vi "UpdateDialog.vi"(8 "error in (no error)":errorcluster, 9 "Engine in":refnum<class "Engine.lvclass">, 11 "Highscore in":refnum<class "HighscoreDialog.lvclass">) -> (0 "error out":errorcluster, 1 "Engine out":refnum<class "Engine.lvclass">, 3 "Highscore out":refnum<class "HighscoreDialog.lvclass">)   [LabVIEW 2019, in "RT_Game.lvlib" / "HighscoreDialog.lvclass"]
uses:
  HighscoreDialog.lvclass
  C:/Users/FreshBob/Dropbox/VIs/myRIO_GameConsole/RT/RT_Game/GameObject/GameObject.lvclass
  Engine/Engine.lvclass
  GameObject/GameObject.lvclass/GameObject.ctl
  GameObject/Read IsActive.vi
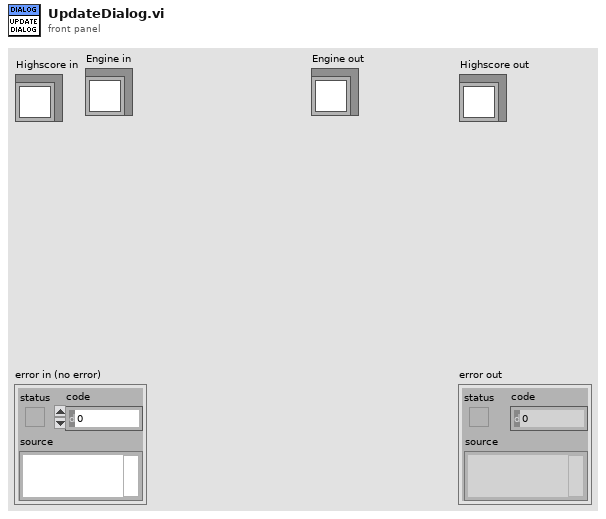
[diagram p1: front panel]
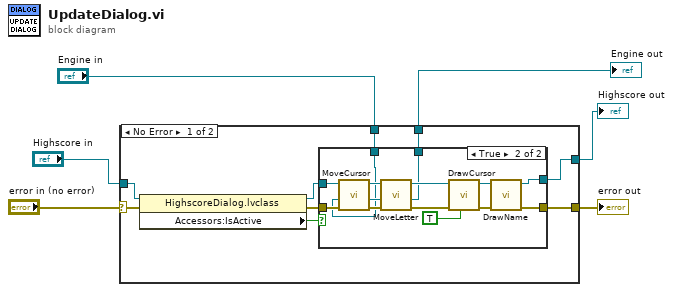
[diagram p0: block diagram]
diagram:
  n1 = case shown="No Error" "error in (no error)" {
    selector: "error in (no error)" -> [w15 w35]
    tunnel: [w13 w35] -> w5
    tunnel: [w14 w34] -> w3
    tunnel: "Highscore in" -> [w11 w34]
    tunnel: "Engine in" -> [w8 w33]
    tunnel: [w7 w33] -> w1
    frame No Error {
      n2 = property class="HighscoreDialog.lvclass"(reference=w11, error in=w15) -> (reference out=w10:refnum<class "HighscoreDialog.lvclass">, error out=w12:errorcluster, "Accessors:IsActive"=w9:bool)
      n3 = case shown="True" w9 {
        tunnel: w12 -> [w17 w32]
        tunnel: w10 -> [w18 w30]
        tunnel: [w18 w23] -> w14
        tunnel: [w17 w22] -> w13
        tunnel: w8 -> [w16 w19]
        tunnel: [w16 w21] -> w7
        frame False {
        }
        frame True {
          n4 = call "MoveCursor.vi"("error in (no error)"=w32, "Engine in"=w19, "Highscore in"=w30) -> ("error out"=w31:errorcluster, "Engine out"=w20:refnum<class "Engine.lvclass">, "Highscore out"=w28:refnum<class "HighscoreDialog.lvclass">)  [unwired: 6 in]
          n5 = call "MoveLetter.vi"("error in (no error)"=w31, "Engine in"=w20, "Highscore in"=w28) -> ("error out"=w29:errorcluster, "Engine out"=w21:refnum<class "Engine.lvclass">, "Highscore out"=w26:refnum<class "HighscoreDialog.lvclass">)  [unwired: 6 in]
          n6 = call "DrawCursor.vi"("Visible?"=TRUE, "error in (no error)"=w29, "Highscore in"=w26) -> ("error out"=w27:errorcluster, "Highscore out"=w24:refnum<class "HighscoreDialog.lvclass">)  [unwired: 7 in]
          n7 = call "DrawName.vi"("error in (no error)"=w27, "Highscore in"=w24) -> ("error out"=w22:errorcluster, "Highscore out"=w23:refnum<class "HighscoreDialog.lvclass">)  [unwired: 8 in]
        }
      }
    }
    frame Error {
    }
  }
  "error out" <- w5
  "Highscore out" <- w3
  "Engine out" <- w1
